vi "nPr_Sub_VI.vi"(10 "n 2":i32, 11 "n":i32) -> (3 "Numeric":dbl)   [LabVIEW 2024]
uses:
  <vilib>/gmath/NI_Gmath.lvlib
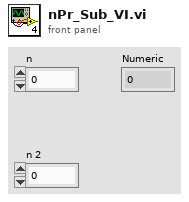
[diagram p1: front panel]
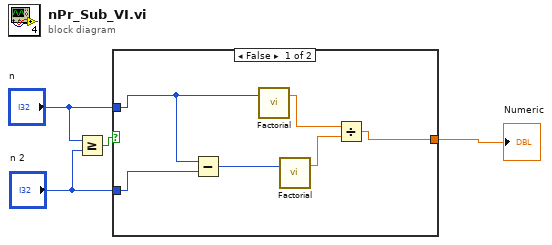
[diagram p0: block diagram]
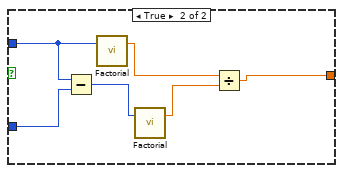
[diagram p2: hidden frame]
diagram:
  n1 = Greater Or Equal?(x="n", y="n 2") -> (x >= y?=w1:bool)
  n2 = case shown="False" w1 {
    tunnel: "n" -> [w10 w16]
    tunnel: "n 2" -> [w9 w15]
    tunnel: [w5 w11] -> w4
    frame False {
      n3 = Subtract(x=w10, y=w9) -> (x-y=w8:i32)
      n4 = call <vilib>:"Factorial.vi"("n"=w10) -> ("n!"=w7:dbl)  [unwired: 2 in]
      n5 = call <vilib>:"Factorial.vi"("n"=w8) -> ("n!"=w6:dbl)  [unwired: 2 in]
      n6 = Divide(x=w7, y=w6) -> (x/y=w5:dbl)
    }
    frame True {
      n7 = Subtract(x=w16, y=w15) -> (x-y=w14:i32)
      n8 = call <vilib>:"Factorial.vi"("n"=w16) -> ("n!"=w13:dbl)  [unwired: 2 in]
      n9 = call <vilib>:"Factorial.vi"("n"=w14) -> ("n!"=w12:dbl)  [unwired: 2 in]
      n10 = Divide(x=w13, y=w12) -> (x/y=w11:dbl)
    }
  }
  "Numeric" <- w4
